vi "17_Control addition.vi"() -> ()   [LabVIEW 2018]
panel:
  out "Answer":dbl
  in  "B":dbl
  in  "A":dbl
  # "Develop a HMI code for two controls and 1 display for simple addition"
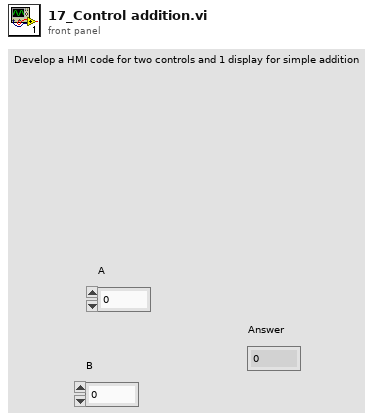
[diagram p1: front panel]
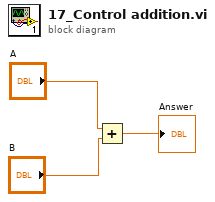
[diagram p0: block diagram]
diagram:
  n1 = Add(x="A", y="B") -> (x+y=→"Answer":dbl)
